vi "DSP_sandbox.vi"() -> ()   [LabVIEW 2016]
uses:
  DSP.lockin/Typedefs/LockinResults.ctl
  DSP.lockin/Typedefs/LockinResult.ctl
  <vilib>/Analysis/4window.llb/windowTd.ctl
  <vilib>/measure/maspectr.llb/Power Spectrum and PSD Export Mode.ctl
  <vilib>/measure/maspectr.llb/FFT Power Spectrum and PSD for N Chan.vi
  <vilib>/Waveform/WDTOps.llb/WDT Waveform to XY Pairs DBL.vi
  lockin/lockin.lvclass
  <vilib>/measure/NI_MAPro.lvlib
  <vilib>/Analysis/NI_AALPro.lvlib
  DSP.lockin/DSP.lockin.lvclass
panel:
  in  "LP config":cluster{"high cutoff freq [Hz]":dbl}={"high cutoff freq [Hz]"=0.45}
  in  "Lockin config":cluster{"TC (s)":dbl, "order":i32}={"TC (s)"=0.5, "order"=2} {"TC (s)" format="%#_13g"}
  in  "FFT config":T3={"averaging parameters"={"averaging mode"=enum."RMS averaging", "weighting mode"=enum."Exponential", "number of averages"=10}, "window"=1, "export mode"=0, "window parameter"=nan, "restart averaging (F)"=FALSE} {"export mode" items=["Power Spectrum", "Power Spectral Density"]; "window" items=["Rectangle"=0, "Hanning"=1, "Hamming"=2, "Blackman-Harris"=3, "Exact Blackman"=4, "Blackman"=5, "Flat Top"=6, "4 Term B-Harris "=7, "7 Term B-Harris"=8, "Low Sidelobe"=9, "Blackman Nuttall"=11, "Triangle"=30, "Bartlett-Hanning"=31, "Bohman"=32, "Parzen"=33, "Welch"=34, "Kaiser"=60, "Dolph-Chebyshev"=61, "Gaussian"=62]; "averaging parameters"."number of averages" min=1}
  in  "Lockin Results":T4
  in  "Reference In":waveform(dbl)[](array[waveform])
  in  "Signal in":waveform(dbl)[](array[waveform])
  out "Signal Out":waveform(dbl)[](array[waveform])
  out "Results (X,Y,R,Theta)":dbl[][](array[numeric])
  out "PS Chart":dbl[][](graph)=[[-1411.497616925462, -1404.3790029743438, -1413.0961920610762, -1418.6418791322994, -1413.136726104145, -1413.4151534226191, -1417.9246313001065, -1424.6072395567076]]
  out "averaging done":bool=TRUE
  out "averages\ncompleted":dbl=8319.0
  out "PS dB":cluster{"f0":dbl, "df":dbl, "magnitude":dbl[]}[](graph)
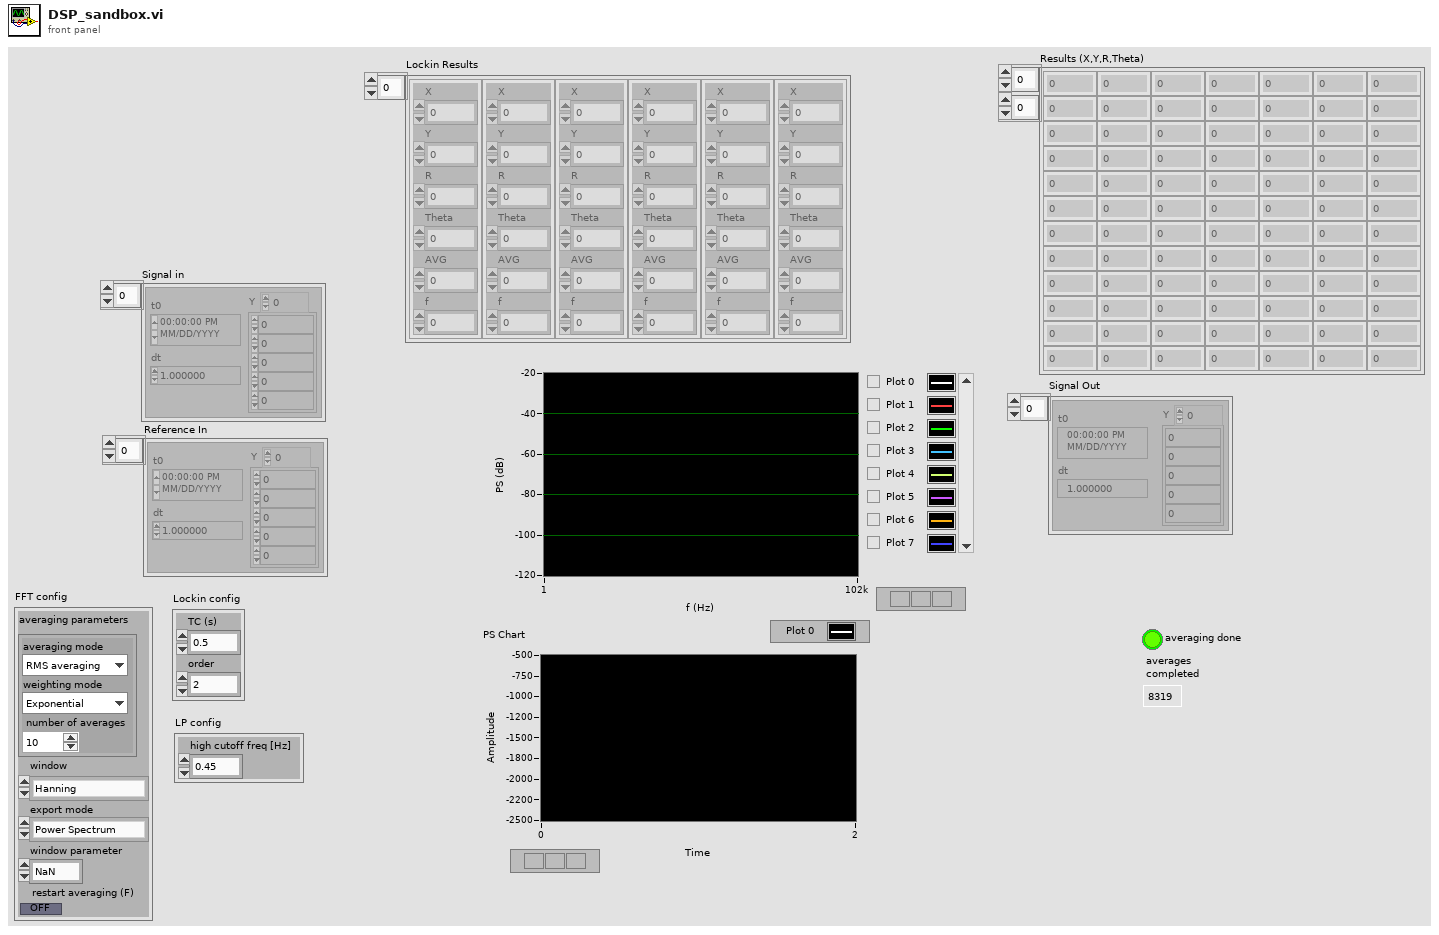
[diagram p1: front panel]
types:
  T1 = typedef "NI_AALPro.lvlib/windowTd.ctl" = u32
  T2 = typedef "NI_MAPro.lvlib/Power Spectrum and PSD Export Mode.ctl" = u16
  T3 = cluster{"averaging parameters":cluster{"averaging mode":enum16{"No averaging", "Vector averaging", "RMS averaging", "Peak hold"}, "weighting mode":enum16{"Linear", "Exponential"}, "number of averages":u32}, "window":T1, "export mode":T2, "window parameter":dbl, "restart averaging (F)":bool}
  T4 = typedef "DSP.lockin.lvclass/LockinResults.ctl" = T5[]
  T5 = typedef "DSP.lockin.lvclass/LockinResult.ctl" = cluster{"X":dbl, "Y":dbl, "R":dbl, "Theta":dbl, "AVG":dbl, "f":dbl}
  T6 = cluster{"averaging mode":enum16{"No averaging", "Vector averaging", "RMS averaging", "Peak hold"}, "weighting mode":enum16{"Linear", "Exponential"}, "number of averages":u32}
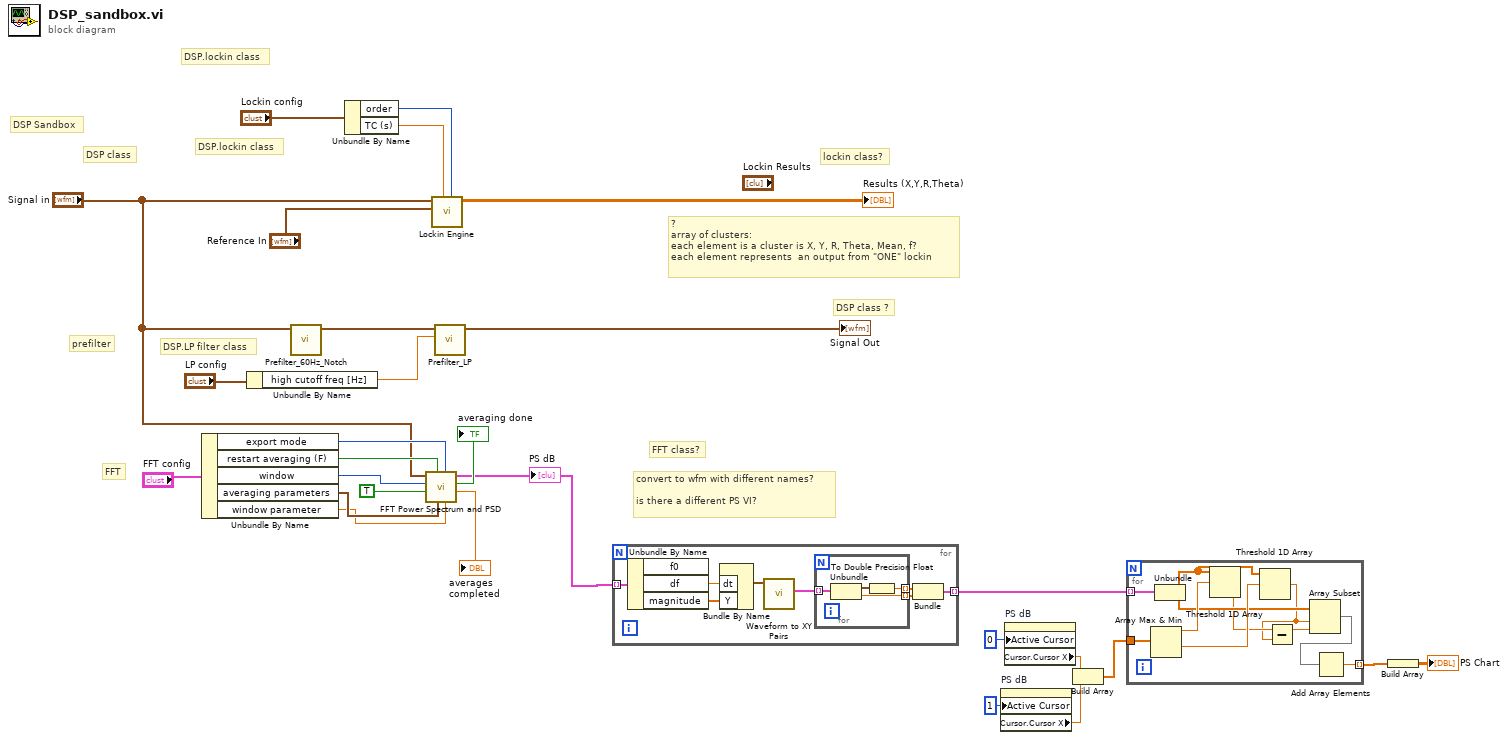
[diagram p0: block diagram]
diagram:
  # "DSP.lockin class"
  # "?\narray of clusters:\neach element is a cluster is X, Y, R, Theta, Mean, f?\neach element represents  an output from \"ONE\" lockin"
  # "convert to wfm with different names?\n\nis there a different PS VI?"
  # "FFT class?"
  # "lockin class?"
  # "DSP class ?"
  # "DSP.LP filter class"
  # "DSP class"
  # "prefilter"
  # "FFT"
  # "DSP.lockin class"
  # "DSP Sandbox"
  n1 = Unbundle By Name("FFT config") -> ("export mode"=w13:T2, "restart averaging (F)"=w12:bool, "window"=w11:T1, "averaging parameters"=w10:T6, "window parameter"=w9:dbl)
  n2 = Unbundle By Name("LP config") -> ("high cutoff freq [Hz]"=w1:dbl)
  n3 = call "Prefilter_60Hz_Notch.vi"("Array"="Signal in") -> ("Array 2"=w28:waveform(dbl)[])  [unwired: 10 in]
  n4 = Unbundle By Name("Lockin config") -> ("order"=w4:i32, "TC (s)"=w3:dbl)
  n5 = call-poly <vilib>:"FFT Power Spectrum and PSD.vi"("window parameter"=w9, "export mode"=w13, "averaging parameters"=w10, "restart averaging (F)"=w12, "dB On (F)"=TRUE, "window"=w11, "time signals"="Signal in") -> ("averages completed"=→"averages\ncompleted":dbl, "averaging done"=→"averaging done":bool, "Power Spectrum / PSD"=w19:cluster{"f0":dbl, "df":dbl, "magnitude":dbl[]}[])  [unwired: 1 in, 1 out]
  "PS dB" <- w19
  n6 = call "Lockin Engine.vi"("order"=w4, "TC (s)"=w3, "Reference In"="Reference In", "Signal in"="Signal in") -> ("Results (X,Y,R,Theta)"=→"Results (X,Y,R,Theta)":dbl[][])  [unwired: 5 in, 2 out]
  n7 = call "Prefilter_LP.vi"("high cutoff freq [Hz]"=w1, "Array"=w28) -> ("Array 2"=→"Signal Out":waveform(dbl)[])  [unwired: 9 in]
  n8 = for {
    tunnel: w19 -> [w34] mode=indexing
    tunnel: [w29] -> w7 mode=indexing
    n9 = Unbundle By Name(w34) -> ("df"=w36:dbl, "magnitude"=w35:dbl[])  [unwired: 1 out]
    n10 = Bundle By Name("dt"=w36, "Y"=w35) -> (w33:waveform(dbl))  [unwired: 1 in]
    n11 = call-poly <vilib>:"Waveform to XY Pairs.vi"("waveform in"=w33) -> ("XY pairs"=w32:cluster{"x":timestamp, "y":dbl}[])  [unwired: 8 in, 2 out]
    n12 = for {
      tunnel: w32 -> [w40] mode=indexing
      tunnel: [w38] -> w30 mode=indexing
      tunnel: [w37] -> w31 mode=indexing
      n13 = Unbundle(w40) -> ("x"=w39:timestamp, "y"=w38:dbl)
      n14 = To Double Precision Float(number=w39) -> (double precision float=w37:dbl)
    }
    n15 = Bundle(w31, w30) -> (w29:cluster{dbl[], dbl[]})  [unwired: 1 in]
  }
  n16 = property on="PS dB" class="WFGraph (strict)"("Active Cursor"=u32 1) -> ("Cursor.Cursor X"=w23:dbl)  [unwired: 2 in, 2 out]
  n17 = property on="PS dB" class="WFGraph (strict)"("Active Cursor"=u32 0) -> ("Cursor.Cursor X"=w24:dbl)  [unwired: 2 in, 2 out]
  n18 = Build Array(w24, w23) -> (w22:dbl[])
  n19 = for {
    tunnel: w7 -> [w51] mode=indexing
    tunnel: w22 -> [w50]
    tunnel: [w42] -> w6 mode=indexing
    n20 = Array Max & Min(array=w50) -> (max value=w49:dbl, min value=w47:dbl)  [unwired: 2 out]
    n21 = Unbundle(w51) -> (w48:dbl[], w46:dbl[])
    n22 = Threshold 1D Array(2:w49, 3:w48) -> (0:w45:dbl)  [unwired: 1 in]
    n23 = Threshold 1D Array(2:w47, 3:w48) -> (0:w44:dbl)  [unwired: 1 in]
    n24 = Subtract(x=w45, y=w44) -> (x-y=w43:dbl)
    n25 = Array Subset(array=w46, index=w44, length=w43) -> (w41:dbl[])
    n26 = Add Array Elements(numeric array=w41) -> (sum=w42:dbl)
  }
  n27 = Build Array(w6) -> (→"PS Chart":dbl[][])
